vi "save_images_2.vi"(6 "p_experiment_path":path, 7 "number of fringes":dbl=4.0, 9 "time (or other uniqe identifier)":string, 10 "images to store (3D pixel array)":u8[][][](array[numeric]), 11 "description (orig./capt.)":string="_original_") -> ()   [LabVIEW 2011]
uses:
  <userlib>/_OpenG.lib/file/file.llb/File Exists - Scalar__ogtk.vi
  global_vars.vi
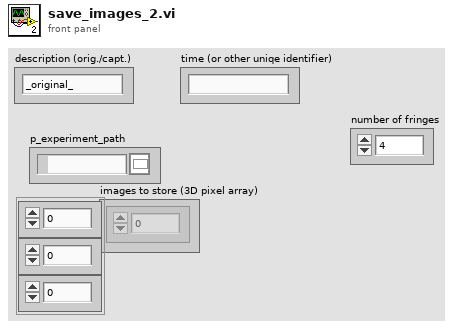
[diagram p1: front panel]
types:
  T1 = typedef "Image Type" = u32
  T2 = typedef "IMAQ Image.ctl" = refnum<image>
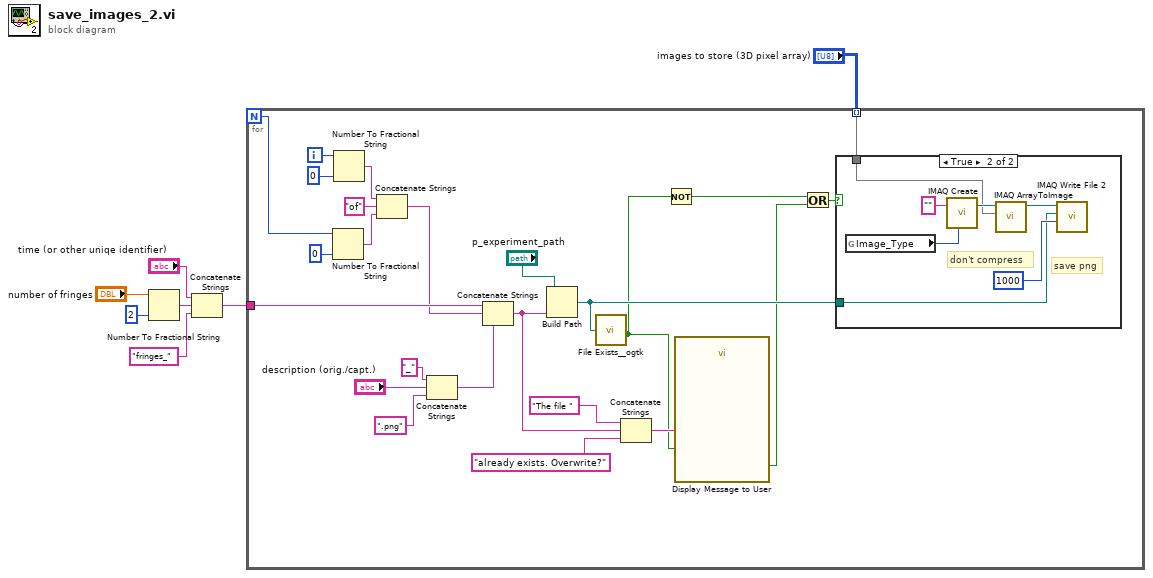
[diagram p0: block diagram]
diagram:
  n1 = Number To Fractional String(number="number of fringes", precision (6)=i16 2) -> (F-format string=w6:string)  [unwired: 2 in]
  n2 = Concatenate Strings("time (or other uniqe identifier)", w6, "fringes_" ("string")) -> (w3:string)
  n3 = for {
    N -> [w30]
    tunnel: w3 -> [w20]
    tunnel: "images to store (3D pixel array)" -> [w23] mode=indexing
    i -> [w26]
    n4 = Number To Fractional String(number=w30, precision (6)=i16 0) -> (F-format string=w28:string)  [unwired: 2 in]
    n5 = Number To Fractional String(number=w26, precision (6)=i16 0) -> (F-format string=w25:string)  [unwired: 2 in]
    n6 = Concatenate Strings(w25, "of" ("string"), w28) -> (w18:string)
    n7 = Concatenate Strings("_" ("string"), "description (orig./capt.)", ".png" ("string")) -> (w17:string)
    n8 = Concatenate Strings(w20, w18, w17) -> (w15:string)
    n9 = Build Path(base path="p_experiment_path", name or relative path=w15) -> (appended path=w19:path)
    n10 = call-poly <userlib>:"File Exists__ogtk.vi"("file path"=w19) -> ("exists"=w9:bool)  [unwired: 6 in, 1 out]
    n11 = Concatenate Strings("The file ", w15, "already exists. Overwrite?" ("string")) -> (w13:string)
    n12 = Not(x=w9) -> (.not. x?=w12:bool)
    n13 = call "Display Message to User"("Enable"=w9, "Message"=w13) -> ("Yes"=w11:bool)  [unwired: 8 in, 1 out]
    n14 = Or(x=w12, y=w11) -> (x .or. y?=w10:bool)
    n15 = case shown="True" w10 {
      tunnel: w23 -> [_ w33]
      tunnel: w19 -> [_ w32]
      frame False {
      }
      frame True {
        # "don't compress"
        # "save png"
        n16 = global read "global_vars.vi" "Image_Type"() -> (w34:T1)
        n17 = call "IMAQ Create"("Image Name"="", "Image Type"=w34) -> ("New Image"=w35:T2)  [unwired: 2 in, 2 out]
        n18 = call "IMAQ ArrayToImage"("Image Pixels (U8)"=w33, "Image"=w35) -> ("Image Out"=w37:T2)  [unwired: 8 in, 1 out]
        n19 = call-poly "IMAQ Write File 2"("Image Quality"=u32 1000, "File Path"=w32, "Image"=w37) -> ()  [unwired: 7 in, 2 out]
      }
    }
  }
